vi "String2Scout.vi"(0 "String":string) -> (2 "Team":u16, 3 "Match":string, 4 "Unique":string, 5 "Team Out":T3, 6 "Auto Out":T2, 7 "Scores Out":T1)   [LabVIEW 2013]
panel:
  out "array":string[][](array[string])
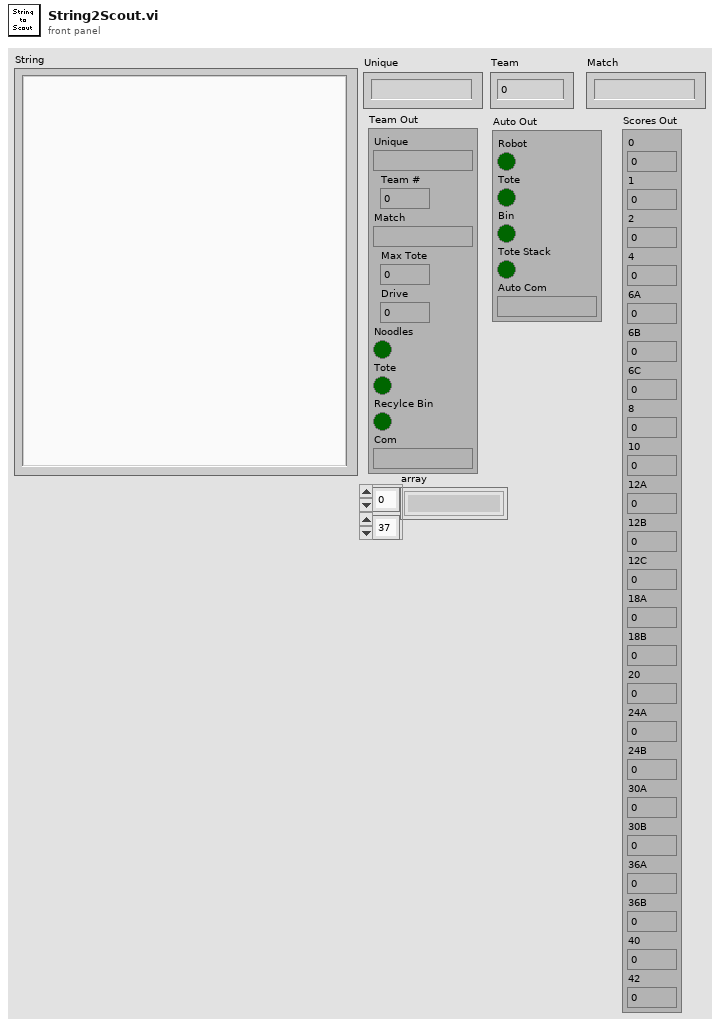
[diagram p1: front panel]
types:
  T1 = cluster{"0":u8, "1":u8, "2":u8, "4":u8, "6A":u8, "6B":u8, "6C":u8, "8":u8, "10":u8, "12A":u8, "12B":u8, "12C":u8, "18A":u8, "18B":u8, "20":u8, "24A":u8, "24B":u8, "30A":u8, "30B":u8, "36A":u8, "36B":u8, "40":u8, "42":u8}
  T2 = cluster{"Robot":bool, "Tote":bool, "Bin":bool, "Tote Stack":bool, "Auto Com":string}
  T3 = cluster{"Unique":string, "Team #":u16, "Match":string, "Max Tote":u8, "Drive":u16, "Noodles":bool, "Tote":bool, "Recylce Bin":bool, "Com":string}
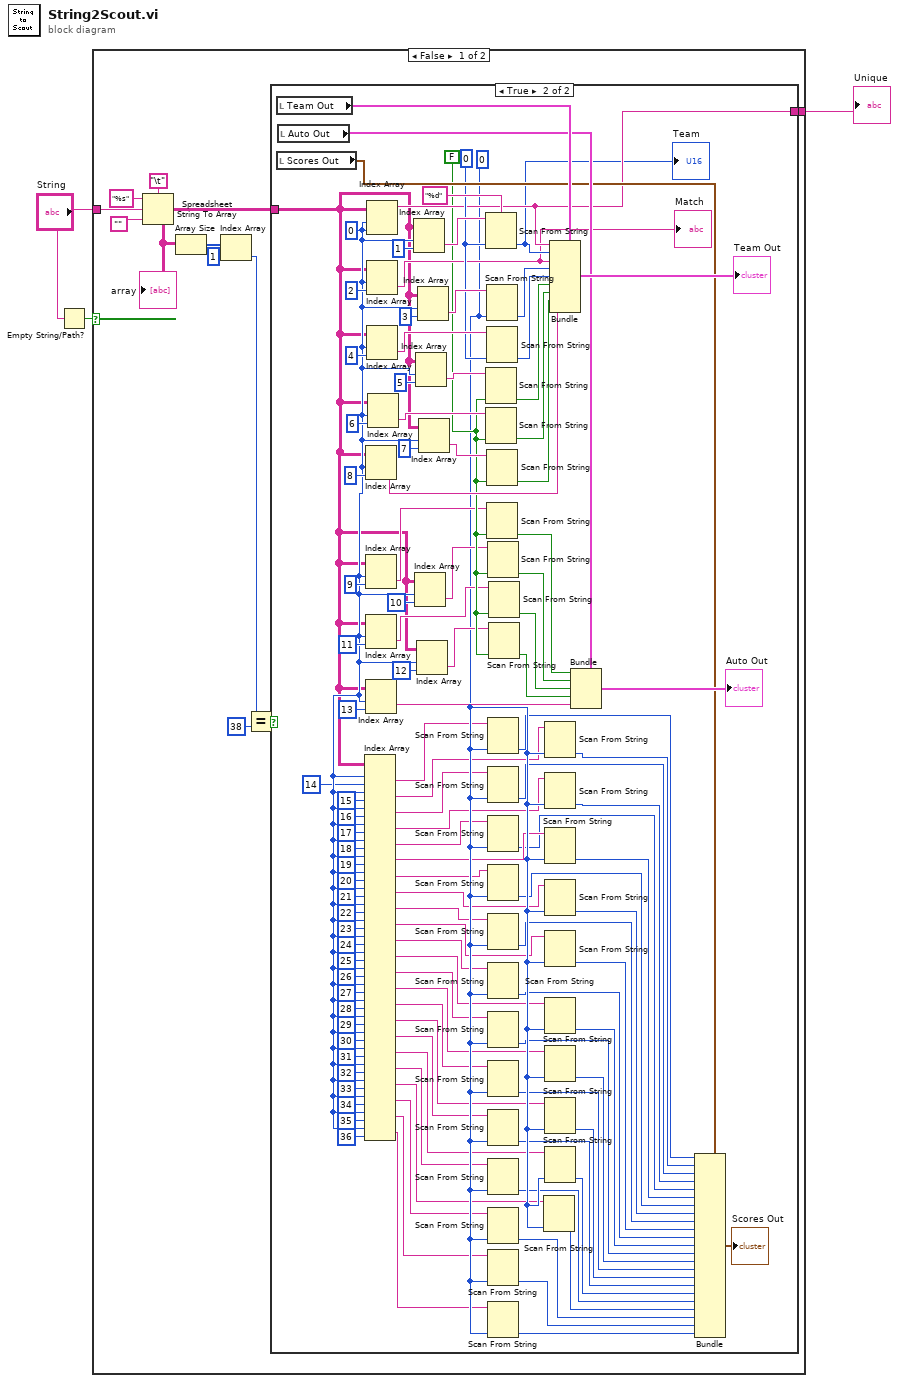
[diagram p0: block diagram]
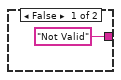
[diagram p2: hidden frame]
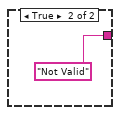
[diagram p3: hidden frame]
diagram:
  n1 = Empty String/Path?(string/path="String") -> (empty?=w2:bool)
  n2 = case shown="False" w2 {
    tunnel: "String" -> [w12 _]
    tunnel: [w10 "Not Valid"] -> w1
    frame False {
      n3 = Spreadsheet String To Array(delimiter (Tab)="\t", format string="%s", spreadsheet string=w12, array type (2D Dbl)="") -> (array=w9:string[][])
      "array" <- w9
      n4 = Array Size(array=w9) -> (size(s)=w8:i32[])
      n5 = Index Array(array=w8, index=1) -> (element=w6:i32)
      n6 = Equal?(x=w6, y=38) -> (x = y?=w4:bool)
      n7 = case shown="True" w4 {
        tunnel: ["Not Valid" w105] -> w10
        tunnel: w9 -> [_ w17]
        frame False {
        }
        frame True {
          w96 = FALSE
          w111 = u16 0
          w86 = u8 0
          w87 = 0 ("disabled index (col)")
          n8 = local read "Team Out"() -> (w130:T3)
          n9 = local read "Scores Out"() -> (w128:T1)
          n10 = local read "Auto Out"() -> (w129:T2)
          n11 = Index Array(array=w17, index (row) #1=w87, index (col) #1=14 ("index (col)"), index (row) #2=w87, index (col) #2=15 ("index (col)"), index (row) #3=w87, index (col) #3=16 ("index (col)"), index (row) #4=w87, index (col) #4=17 ("index (col)"), index (row) #5=w87, index (col) #5=18 ("index (col)"), index (row) #6=w87, index (col) #6=19 ("index (col)"), index (row) #7=w87, index (col) #7=20 ("index (col)"), index (row) #8=w87, index (col) #8=21 ("index (col)"), index (row) #9=w87, index (col) #9=22 ("index (col)"), index (row) #10=w87, index (col) #10=23 ("index (col)"), index (row) #11=w87, index (col) #11=24 ("index (col)"), index (row) #12=w87, index (col) #12=25 ("index (col)"), index (row) #13=w87, index (col) #13=26 ("index (col)"), index (row) #14=w87, index (col) #14=27 ("index (col)"), index (row) #15=w87, index (col) #15=28 ("index (col)"), index (row) #16=w87, index (col) #16=29 ("index (col)"), index (row) #17=w87, index (col) #17=30 ("index (col)"), index (row) #18=w87, index (col) #18=31 ("index (col)"), index (row) #19=w87, index (col) #19=32 ("index (col)"), index (row) #20=w87, index (col) #20=33 ("index (col)"), index (row) #21=w87, index (col) #21=34 ("index (col)"), index (row) #22=w87, index (col) #22=35 ("index (col)"), index (row) #23=w87, index (col) #23=36 ("index (col)")) -> (element #1=w62:string, element #2=w61:string, element #3=w60:string, element #4=w59:string, element #5=w58:string, element #6=w57:string, element #7=w56:string, element #8=w55:string, element #9=w54:string, element #10=w53:string, element #11=w52:string, element #12=w51:string, element #13=w50:string, element #14=w49:string, element #15=w48:string, element #16=w47:string, element #17=w46:string, element #18=w45:string, element #19=w16:string, element #20=w44:string, element #21=w43:string, element #22=w42:string, element #23=w41:string)
          n12 = Index Array(array=w17, index (row)=w87, index (col)=8) -> (element=w106:string)
          n13 = Index Array(array=w17, index (row)=w87, index (col)=9 ("disabled index (col)")) -> (element=w91:string)
          n14 = Index Array(array=w17, index (row)=w87, index (col)=11 ("disabled index (col)")) -> (element=w89:string)
          n15 = Index Array(array=w17, index (row)=w87, index (col)=13 ("disabled index (col)")) -> (element=w102:string)
          n16 = Index Array(array=w17, index (row)=w87, index (col)=w87) -> (element=w105:string)
          n17 = Index Array(array=w17, index (row)=w87, index (col)=2 ("disabled index (col)")) -> (element=w103:string)
          "Match" <- w103
          n18 = Index Array(array=w17, index (row)=w87, index (col)=4 ("disabled index (col)")) -> (element=w117:string)
          n19 = Index Array(array=w17, index (row)=w87, index (col)=6) -> (element=w114:string)
          n20 = Index Array(array=w17, index (row)=w87, index (col)=1 ("disabled index (col)")) -> (element=w122:string)
          n21 = Index Array(array=w17, index (row)=w87, index (col)=10 ("disabled index (col)")) -> (element=w90:string)
          n22 = Index Array(array=w17, index (row)=w87, index (col)=5 ("disabled index (col)")) -> (element=w115:string)
          n23 = Index Array(array=w17, index (row)=w87, index (col)=12 ("disabled index (col)")) -> (element=w88:string)
          n24 = Index Array(array=w17, index (row)=w87, index (col)=3 ("disabled index (col)")) -> (element=w118:string)
          n25 = Index Array(array=w17, index (row)=w87, index (col)=7) -> (element=w113:string)
          n26 = Scan From String(format string="%d", input string=w122, default 1=w111) -> (output 1=w104:u16)  [unwired: 2 in, 3 out]
          "Team" <- w104
          n27 = Scan From String(input string=w115, default 1=w96) -> (output 1=w109:bool)  [unwired: 3 in, 3 out]
          n28 = Scan From String(input string=w114, default 1=w96) -> (output 1=w108:bool)  [unwired: 3 in, 3 out]
          n29 = Scan From String(input string=w118, default 1=w86) -> (output 1=w110:u8)  [unwired: 3 in, 3 out]
          n30 = Scan From String(input string=w117, default 1=w111) -> (output 1=w112:u16)  [unwired: 3 in, 3 out]
          n31 = Scan From String(input string=w113, default 1=w96) -> (output 1=w107:bool)  [unwired: 3 in, 3 out]
          n32 = Scan From String(input string=w91, default 1=w96) -> (output 1=w95:bool)  [unwired: 3 in, 3 out]
          n33 = Scan From String(input string=w90, default 1=w96) -> (output 1=w94:bool)  [unwired: 3 in, 3 out]
          n34 = Scan From String(input string=w62, default 1=w86) -> (output 1=w36:u8)  [unwired: 3 in, 3 out]
          n35 = Scan From String(input string=w60, default 1=w86) -> (output 1=w34:u8)  [unwired: 3 in, 3 out]
          n36 = Scan From String(input string=w58, default 1=w86) -> (output 1=w32:u8)  [unwired: 3 in, 3 out]
          n37 = Scan From String(input string=w56, default 1=w86) -> (output 1=w30:u8)  [unwired: 3 in, 3 out]
          n38 = Scan From String(input string=w54, default 1=w86) -> (output 1=w28:u8)  [unwired: 3 in, 3 out]
          n39 = Scan From String(input string=w52, default 1=w86) -> (output 1=w26:u8)  [unwired: 3 in, 3 out]
          n40 = Scan From String(input string=w50, default 1=w86) -> (output 1=w24:u8)  [unwired: 3 in, 3 out]
          n41 = Scan From String(input string=w48, default 1=w86) -> (output 1=w22:u8)  [unwired: 3 in, 3 out]
          n42 = Scan From String(input string=w46, default 1=w86) -> (output 1=w20:u8)  [unwired: 3 in, 3 out]
          n43 = Scan From String(input string=w16, default 1=w86) -> (output 1=w18:u8)  [unwired: 3 in, 3 out]
          n44 = Scan From String(input string=w43, default 1=w86) -> (output 1=w38:u8)  [unwired: 3 in, 3 out]
          n45 = Scan From String(input string=w42, default 1=w86) -> (output 1=w39:u8)  [unwired: 3 in, 3 out]
          n46 = Scan From String(input string=w41, default 1=w86) -> (output 1=w40:u8)  [unwired: 3 in, 3 out]
          n47 = Scan From String(input string=w89, default 1=w96) -> (output 1=w93:bool)  [unwired: 3 in, 3 out]
          n48 = Scan From String(input string=w88, default 1=w96) -> (output 1=w92:bool)  [unwired: 3 in, 3 out]
          n49 = Scan From String(input string=w44, default 1=w86) -> (output 1=w37:u8)  [unwired: 3 in, 3 out]
          n50 = Scan From String(input string=w61, default 1=w86) -> (output 1=w35:u8)  [unwired: 3 in, 3 out]
          n51 = Scan From String(input string=w59, default 1=w86) -> (output 1=w33:u8)  [unwired: 3 in, 3 out]
          n52 = Scan From String(input string=w57, default 1=w86) -> (output 1=w31:u8)  [unwired: 3 in, 3 out]
          n53 = Scan From String(input string=w55, default 1=w86) -> (output 1=w29:u8)  [unwired: 3 in, 3 out]
          n54 = Scan From String(input string=w53, default 1=w86) -> (output 1=w27:u8)  [unwired: 3 in, 3 out]
          n55 = Scan From String(input string=w51, default 1=w86) -> (output 1=w25:u8)  [unwired: 3 in, 3 out]
          n56 = Scan From String(input string=w49, default 1=w86) -> (output 1=w23:u8)  [unwired: 3 in, 3 out]
          n57 = Scan From String(input string=w47, default 1=w86) -> (output 1=w21:u8)  [unwired: 3 in, 3 out]
          n58 = Scan From String(input string=w45, default 1=w86) -> (output 1=w19:u8)  [unwired: 3 in, 3 out]
          n59 = Bundle(cluster=w130, "Unique"=w105, "Team #"=w104, "Match"=w103, "Max Tote"=w110, "Drive"=w112, "Noodles"=w109, "Tote"=w108, "Recylce Bin"=w107, "Com"=w106) -> (→"Team Out":T3)
          n60 = Bundle(cluster=w129, "Robot"=w95, "Tote"=w94, "Bin"=w93, "Tote Stack"=w92, "Auto Com"=w102) -> (→"Auto Out":T2)
          n61 = Bundle(cluster=w128, "0"=w36, "1"=w35, "2"=w34, "4"=w33, "6A"=w32, "6B"=w31, "6C"=w30, "8"=w29, "10"=w28, "12A"=w27, "12B"=w26, "12C"=w25, "18A"=w24, "18B"=w23, "20"=w22, "24A"=w21, "24B"=w20, "30A"=w19, "30B"=w18, "36A"=w37, "36B"=w38, "40"=w39, "42"=w40) -> (→"Scores Out":T1)
        }
      }
    }
    frame True {
    }
  }
  "Unique" <- w1
